vi "P9374AEasilyUse_sweepDC.vi"() -> ()   [LabVIEW 2016]
uses:
  <vilib>/Utility/file.llb/Write Delimited Spreadsheet (DBL).vi
  <instrlib>/Agilent NA/Agilent NA.lvlib
panel:
  in  "File type":string=".txt"
  in  "Filename":string="test"
  in  "Path":path=path "P:/"
  in  "Start":i32
  in  "Step Size":dbl=0.05 format="%#_13g"
  in  "Lockin channel":i32
  in  "Steps":i32
  out "error out":errorcluster
  out "S Parameter":string="S21"
  in  "S-Paramter":u16(ring) items=["S11", "S12", "S21", "S22"]
  in  "Data Points":i32=2048 format="%.3g"
  in  "Measurement":string="Measurement1"
  in  "Averaging Factor":i32=30
  in  "Milliseconds to wait for averaging":u32=10000
  out "Graph":dbl[](graph)
  in  "Averaging":bool=TRUE
  in  "Start Frequency":dbl=300000000.0 format="%#_13p"
  in  "Stop Frequency":dbl=10000000000.0 format="%#_13p"
  in  "Source Power (dBm)":dbl=-40.0 format="%#_13g"
  in  "Channel":string="Channel1"
  in  "resource string":string="PXI10::CHASSIS1::SLOT1::FUNC0::INSTR" caption="resource name"
  # "Warning: Before running this VI, open the I/O interface first!!!!!!"
  # "Settings"
  # "Data Acquizition"
  # "Usually do not need to change."
  # "for both ports"
  # "If True"
  # "Default: 2048"
  # "Wait time should be long enough \nfor VNA to finish averaging."
  # "Set the S-parameter you want to take\nS11: Source1, Receiver1\nS12: Source2, Receiver1\nS21: Source1, Receiver2\nS22: Source2, Receiver2"
  # "Other things need to be set from front panel:\nIF band width (always default)"
  # "DC voltage sweep setting"
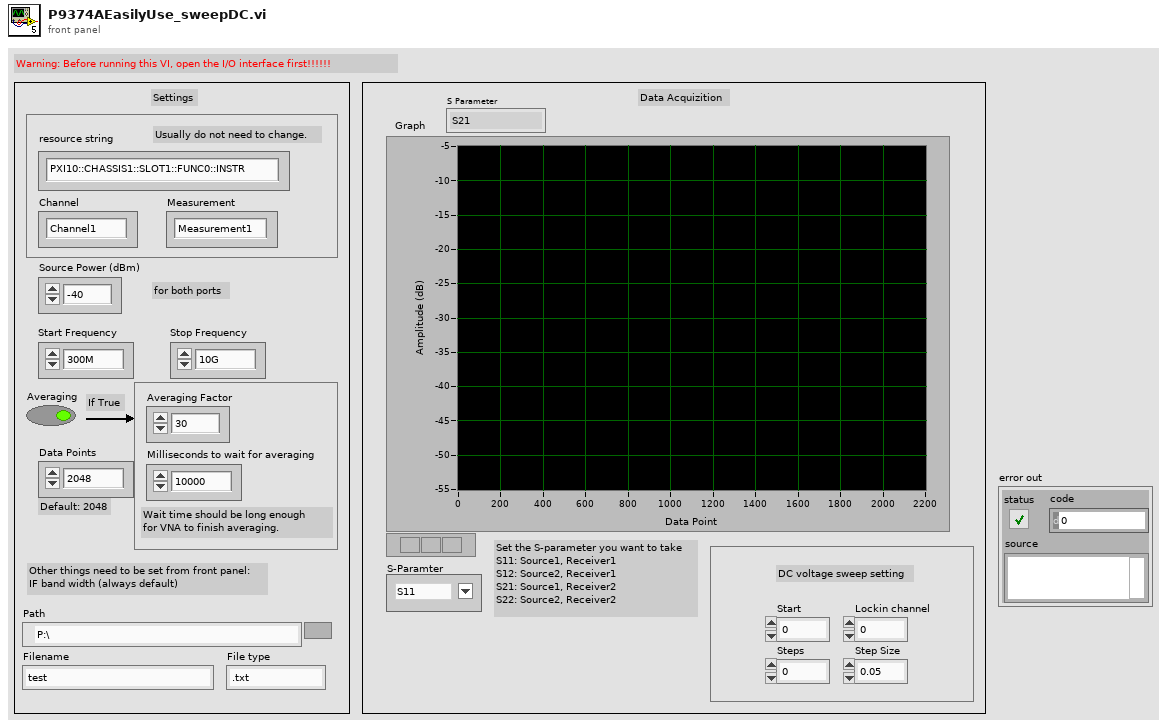
[diagram p1: front panel]
types:
  T1 = cluster{"AO amp (V)":dbl[], "AO DC (V)":dbl[], "AO f (Hz)":dbl[], "AO phi (deg)":dbl[], "function":enum16{"Sine Wave", "Triangle Wave", "Square Wave", "Sawtooth Wave"}[]}
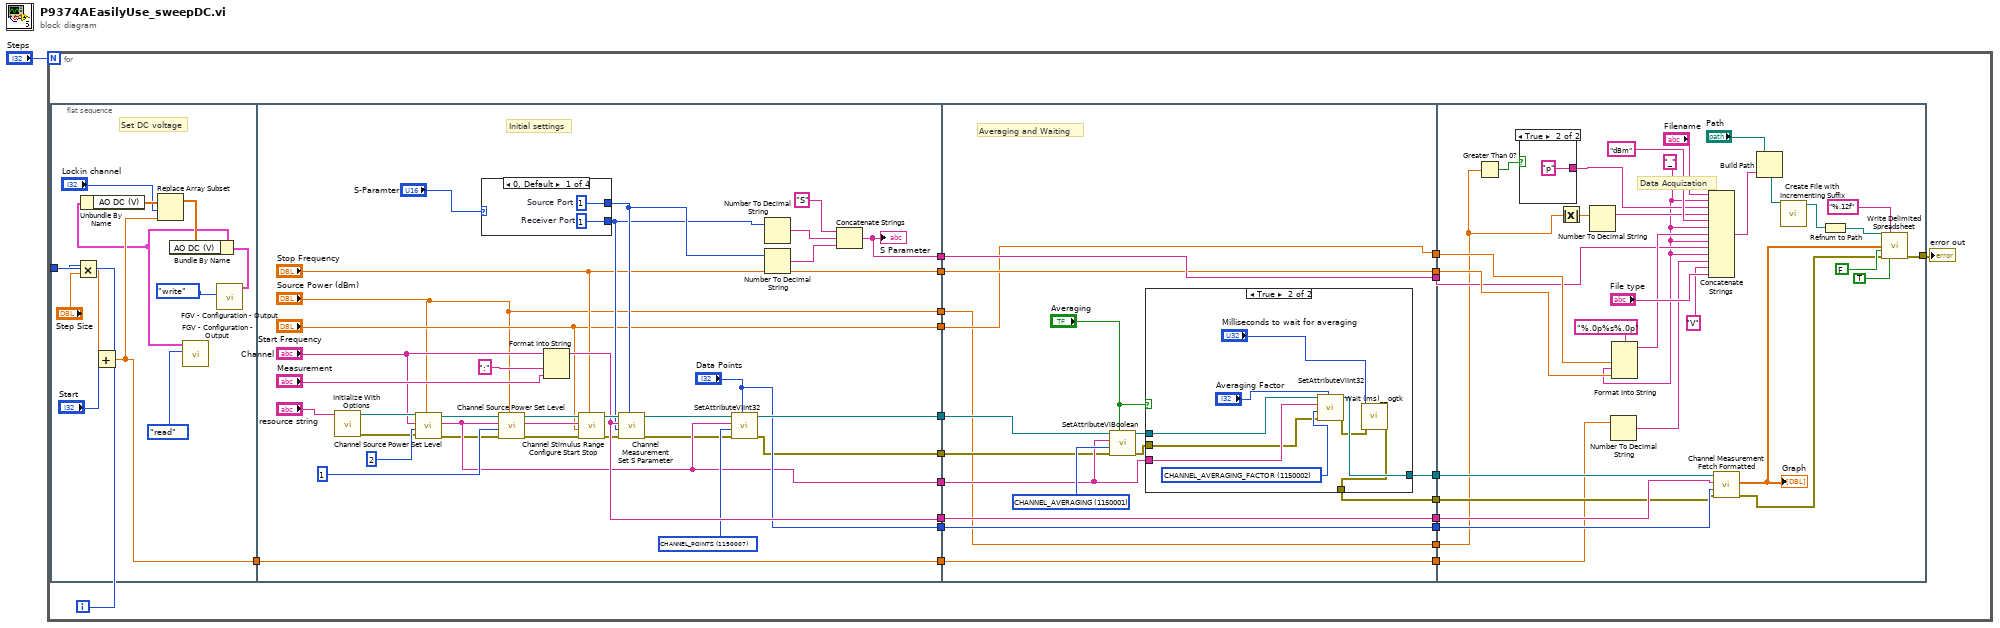
[diagram p0: block diagram]
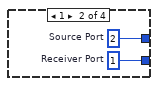
[diagram p2: hidden frame]
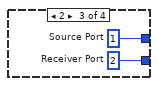
[diagram p3: hidden frame]
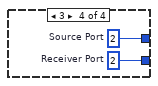
[diagram p4: hidden frame]
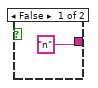
[diagram p6: hidden frame]
diagram:
  n1 = for {
    N: "Steps" -> [_]
    i -> [w11]
    n2 = flat-sequence {
      tunnel: w11 -> [w35]
      tunnel: [w29] -> w10
      tunnel: [w60] -> w23
      tunnel: ["Channel"] -> w22
      tunnel: [w58] -> w21
      tunnel: ["Data Points"] -> w20
      tunnel: [w47] -> w19
      tunnel: [w40] -> w18
      tunnel: w10 -> [w39]
      tunnel: [w39] -> w9
      tunnel: ["Stop Frequency"] -> w6
      tunnel: ["Start Frequency"] -> w4
      tunnel: ["Source Power (dBm)"] -> w2
      tunnel: w23 -> [w84]
      tunnel: w22 -> [w86]
      tunnel: w21 -> [w89]
      tunnel: [w85] -> w17
      tunnel: [w84] -> w16
      tunnel: [w83] -> w15
      tunnel: w20 -> [w83]
      tunnel: w19 -> [w82]
      tunnel: [w80] -> w14
      tunnel: w18 -> [w79]
      tunnel: [w79] -> w13
      tunnel: w9 -> [w78]
      tunnel: [w78] -> w8
      tunnel: [w77] -> w7
      tunnel: w6 -> [w77]
      tunnel: [w76] -> w5
      tunnel: w4 -> [w76]
      tunnel: [w75] -> w3
      tunnel: w2 -> [w75]
      tunnel: w17 -> [w133]
      tunnel: w16 -> [w132]
      tunnel: w15 -> [w131]
      tunnel: w14 -> [w130]
      tunnel: w13 -> [w109]
      tunnel: [w124] -> w12
      tunnel: w8 -> [w104]
      tunnel: w7 -> [w112]
      tunnel: w5 -> [w111]
      tunnel: w3 -> [w106]
      frame #0 {
        # "Set DC voltage"
        n3 = Multiply(x=w35, y="Step Size") -> (x*y=w32:dbl)
        n4 = Add(x=w32, y="Start") -> (x+y=w29:dbl)
        n5 = call <userlib>:"FGV - Configuration - Output.vi"("Function"=enum16{"write", "read"}."read") -> ("Channels: AO 2"=w24:T1)  [unwired: 5 in, 1 out]
        n6 = Unbundle By Name(w24) -> ("AO DC (V)"=w30:dbl[])
        n7 = Replace Array Subset(array=w30, new element=w29, index="Lockin channel") -> (w27:dbl[])
        n8 = Bundle By Name(cluster=w24, "AO DC (V)"=w27) -> (w26:T1)
        n9 = call <userlib>:"FGV - Configuration - Output.vi"("Function"=enum16{"write", "read"}."write", "Channels: AO"=w26) -> ()  [unwired: 4 in, 2 out]
      }
      frame #1 {
        w57 = u32 1150007 items=["CHANNEL_AVERAGING_FACTOR"=1150002, "CHANNEL_MEASUREMENT_ELECTRICAL_DELAY_MEDIUM"=1150178, "CHANNEL_MEASUREMENT_ELECTRICAL_DELAY_UNITS"=1150175, "CHANNEL_MEASUREMENT_FORMAT"=1150014, "CHANNEL_MEASUREMENT_LIMIT_NUMBER"=1150020, "CHANNEL_MEASUREMENT_TIME_DOMAIN_GATING_SHAPE"=1150140, "CHANNEL_MEASUREMENT_TIME_DOMAIN_GATING_TYPE"=1150144, "CHANNEL_MEASUREMENT_TIME_DOMAIN_PARAMETERS"=1150137, "CHANNEL_MEASUREMENT_TIME_DOMAIN_TRANSFORM_MODE"=1150147, "CHANNEL_MEASUREMENT_TRACE_MATH"=1150017, "CHANNEL_POINTS"=1150007, "CHANNEL_SWEEP_MODE"=1150009, "CHANNEL_SWEEP_TYPE"=1150012, "CHANNEL_TRIGGER_MODE"=1150013, "DISPLAY_ARRANGE_WINDOWS"=1150181, "SYSTEM_TIME_OUT_MILLISECONDS"=1150040, "TRIGGER_SOURCE"=1150042, "WINDOW_SIZE"=1150133, "WINDOW_TABLE"=1150134] ("AttributeID")
        # "Initial settings"
        n10 = call <instrlib>:"Initialize With Options.vi"("resource string"="resource string") -> ("error out"=w51:errorcluster, "instrument handle out"=w55:refnum<k15>)  [unwired: 9 in]
        n11 = call <instrlib>:"Channel Source Power Set Level.vi"("Val"="Source Power (dBm)", "error in (no error)"=w51, "PortVal"=2 ("Source Port"), "RepCapIdentifier"="Channel", "instrument handle"=w55) -> ("error out"=w50:errorcluster)  [unwired: 5 in, 1 out]
        n12 = case shown="0, Default" "S-Paramter" {
          tunnel: [w68 w70 w72 w74] -> w42
          tunnel: [w67 w69 w71 w73] -> w41
          frame 0, Default {
            w67 = 1  # Receiver Port
            w68 = 1  # Source Port
          }
          frame 1 {
            w69 = 1  # Receiver Port
            w70 = 2  # Source Port
          }
          frame 2 {
            w71 = 2  # Receiver Port
            w72 = 1  # Source Port
          }
          frame 3 {
            w73 = 2  # Receiver Port
            w74 = 2  # Source Port
          }
        }
        n13 = call <instrlib>:"Channel Source Power Set Level.vi"("Val"="Source Power (dBm)", "error in (no error)"=w50, "PortVal"=1 ("Source Port"), "RepCapIdentifier"="Channel", "instrument handle"=w55) -> ("error out"=w52:errorcluster, "instrument handle out"=w64:refnum<k15>)  [unwired: 5 in]
        n14 = Format Into String(initial string="Channel", ":", "Measurement") -> (resulting string=w60:string)  [unwired: 2 in, 1 out]
        n15 = call <instrlib>:"Channel Stimulus Range Configure Start Stop.vi"("StopVal"="Stop Frequency", "error in (no error)"=w52, "StartVal"="Start Frequency", "RepCapIdentifier"="Channel", "instrument handle"=w64) -> ("error out"=w49:errorcluster, "instrument handle out"=w63:refnum<k15>)  [unwired: 5 in]
        n16 = call <instrlib>:"Channel Measurement Set S Parameter.vi"("NewSourcePortVal"=w42, "error in (no error)"=w49, "NewReceiverPortVal"=w41, "RepCapIdentifier"=w60, "instrument handle"=w63) -> ("error out"=w48:errorcluster, "instrument handle out"=w59:refnum<k15>)  [unwired: 5 in]
        n17 = call <instrlib>:"SetAttributeViInt32.vi"("AttributeValue"="Data Points", "error in (no error)"=w48, "AttributeID"=w57, "RepCapIdentifier"="Channel", "instrument handle"=w59) -> ("error out"=w47:errorcluster, "instrument handle out"=w58:refnum<k15>)  [unwired: 5 in]
        n18 = Number To Decimal String(number=w41) -> (decimal integer string=w44:string)  [unwired: 1 in]
        n19 = Number To Decimal String(number=w42) -> (decimal integer string=w43:string)  [unwired: 1 in]
        n20 = Concatenate Strings("S" ("string"), w44, w43) -> (w40:string)
        "S Parameter" <- w40
      }
      frame #2 {
        w90 = u32 1150001 items=["CHANNEL_AVERAGING"=1150001, "CHANNEL_CORRECTION"=1150003, "CHANNEL_MEASUREMENT_LIMIT_ENABLE"=1150018, "CHANNEL_MEASUREMENT_MARKER_ENABLED"=1150022, "CHANNEL_MEASUREMENT_MARKER_MARKER_TRACK_ENABLED"=1150023, "CHANNEL_MEASUREMENT_SMOOTHING"=1150015, "CHANNEL_MEASUREMENT_TIME_DOMAIN_COUPLING_STATE"=1150136, "CHANNEL_MEASUREMENT_TIME_DOMAIN_GATING_ENABLE"=1150139, "CHANNEL_MEASUREMENT_TIME_DOMAIN_TRANSFORM_ENABLE"=1150146, "CHANNEL_MEASUREMENT_TRACE_ENABLE_TRACE_MAX"=1150182, "CHANNEL_PORT_EXTENSION_STATUS"=1150008, "CHANNEL_SOURCEPOWER_COUPLING"=1150031, "CHANNEL_SWEEP_TIME_AUTO"=1150011, "DISPLAY_ENABLED"=1150036, "GUIDED_CALIBRATION_ADVANCED_E_CAL_AUTO_ORIENTATION"=1150116, "SIMULATE"=1050005, "SYSTEM_POWER_ENABLED"=1150184, "SYSTEM_TRACE_ENABLED"=1150041, "WINDOW_STATE"=1150183, "WINDOW_TITLE_STATE"=1150132] ("AttributeID")
        # "Averaging and Waiting"
        n21 = call <instrlib>:"SetAttributeViBoolean.vi"("AttributeValue (Off)"="Averaging", "error in (no error)"=w82, "AttributeID"=w90, "RepCapIdentifier"=w86, "instrument handle"=w89) -> ("error out"=w81:errorcluster, "instrument handle out"=w87:refnum<k15>)  [unwired: 5 in]
        n22 = case shown="True" "Averaging" {
          tunnel: w87 -> [w92 w100]
          tunnel: w86 -> [_ w98]
          tunnel: [w92 w97] -> w85
          tunnel: w81 -> [w91 w96]
          tunnel: [w91 w94] -> w80
          frame False {
          }
          frame True {
            w99 = u32 1150002 items=["CHANNEL_AVERAGING_FACTOR"=1150002, "CHANNEL_MEASUREMENT_ELECTRICAL_DELAY_MEDIUM"=1150178, "CHANNEL_MEASUREMENT_ELECTRICAL_DELAY_UNITS"=1150175, "CHANNEL_MEASUREMENT_FORMAT"=1150014, "CHANNEL_MEASUREMENT_LIMIT_NUMBER"=1150020, "CHANNEL_MEASUREMENT_TIME_DOMAIN_GATING_SHAPE"=1150140, "CHANNEL_MEASUREMENT_TIME_DOMAIN_GATING_TYPE"=1150144, "CHANNEL_MEASUREMENT_TIME_DOMAIN_PARAMETERS"=1150137, "CHANNEL_MEASUREMENT_TIME_DOMAIN_TRANSFORM_MODE"=1150147, "CHANNEL_MEASUREMENT_TRACE_MATH"=1150017, "CHANNEL_POINTS"=1150007, "CHANNEL_SWEEP_MODE"=1150009, "CHANNEL_SWEEP_TYPE"=1150012, "CHANNEL_TRIGGER_MODE"=1150013, "DISPLAY_ARRANGE_WINDOWS"=1150181, "SYSTEM_TIME_OUT_MILLISECONDS"=1150040, "TRIGGER_SOURCE"=1150042, "WINDOW_SIZE"=1150133, "WINDOW_TABLE"=1150134] ("AttributeID")
            n23 = call <instrlib>:"SetAttributeViInt32.vi"("AttributeValue"="Averaging Factor", "error in (no error)"=w96, "AttributeID"=w99, "RepCapIdentifier"=w98, "instrument handle"=w100) -> ("error out"=w95:errorcluster, "instrument handle out"=w97:refnum<k15>)  [unwired: 5 in]
            n24 = call <userlib>:"Wait (ms)__ogtk.vi"("error in (no error)"=w95, "milliseconds to wait"="Milliseconds to wait for averaging") -> ("error out"=w94:errorcluster)  [unwired: 8 in, 1 out]
          }
        }
      }
      frame #3 {
        w105 = "_" ("string")
        # "Data Acquization"
        n25 = Greater Than 0?(x=w106) -> (x > 0?=w113:bool)
        n26 = case shown="True" w113 {
          tunnel: ["n" "p"] -> w114
          frame False {
          }
          frame True {
          }
        }
        n27 = Absolute Value(x=w106) -> (abs(x)=w118:dbl)
        n28 = Number To Decimal String(number=w118) -> (decimal integer string=w117:string)  [unwired: 1 in]
        n29 = Number To Decimal String(number=w104) -> (decimal integer string=w103:string)  [unwired: 1 in]
        n30 = Format Into String(format string="%.0p%s%.0p", w111, w105, w112) -> (resulting string=w115:string)  [unwired: 2 in, 1 out]
        n31 = Concatenate Strings("Filename", w105, w114, w117, "dBm" ("string"), w105, w115, w105, w109, w105, w103, "V" ("string"), "File type") -> (w122:string)
        n32 = call <instrlib>:"Channel Measurement Fetch Formatted.vi"("error in (no error)"=w130, "RetValBufferSize"=w131, "RepCapIdentifier"=w132, "instrument handle"=w133) -> ("error out"=w125:errorcluster, "RetVal"=w126:dbl[])  [unwired: 4 in, 2 out]
        "Graph" <- w126
        n33 = Build Path(base path="Path", name or relative path=w122) -> (appended path=w110:path)
        n34 = call <vilib>:"Create File with Incrementing Suffix.vi"("file path"=w110) -> ("refnum out"=w108:refnum<file>)  [unwired: 8 in, 2 out]
        n35 = Refnum to Path(1:w108) -> (0:w107:path)
        n36 = call-poly <vilib>:"Write Delimited Spreadsheet.vi"("file path (dialog if empty)"=w107, "format (%.3f)"="%.12f", "1D data"=w126, "append to file? (new file:F)"=FALSE, "error in (no error)"=w125, "transpose? (no:F)"=TRUE) -> ("error out"=w124:errorcluster)  [unwired: 8 in, 1 out]
      }
    }
    "error out" <- w12
  }
